vi "Robot Global Data.vi"() -> ()   [LabVIEW 2013]
doc: "This global VI can contain as many global variables as you need. Place a control on the panel, give it a good name. To read or write to it from a VI, drag the icon to the diagram of that VI. You can also drag from the project. Click on the node to change which global you access. You shouldn't have multiple locations writing to a global or it will cause a race-condition."
uses:
  <vilib>/Rock Robotics/WPI/Camera/WPI_CameraImageSize.ctl
  <vilib>/Rock Robotics/WPI/DriverStation/WPI_DriverStationRobotMode2.ctl
  Systems/DriverStation/DriverStation.lvclass
  Systems/Shifter/Shifter.lvclass
  Systems/GrabberArms/GrabberArms.lvclass
  Systems/GrabberWheels/GrabberWheels.lvclass
  Systems/Catapult/Catapult.lvclass
  Systems/Compressor/Compressor.lvclass
  Systems/DriveMotors/DriveMotors.lvclass
  Systems/Blocker/Blocker.lvclass
panel:
  out "Low Goal Auto":bool
  out "Catapult Auto":bool
  out "Block Auto":bool
  in  "Power":dbl
  in  "Time to Drive":u32
  out "Trim Left(T) or Right(F)":bool
  in  "Trim":dbl
  in  "Distance to Travel":dbl
  out "AutoMode: Drive Forward and Shoot":bool
  out "Blocker Enabled":bool=TRUE
  out "Catapult Enabled":bool=TRUE
  out "Shifter Enabled":bool=TRUE
  out "Grabber Wheels Enabled":bool=TRUE
  out "Grabber Arms Enabled":bool=TRUE
  out "DML Enabled":bool=TRUE
  out "DMR Enabled":bool=TRUE
  in  "Blocker":refnum<class "Blocker.lvclass">
  out "DMR":refnum<class "DriveMotors.lvclass">
  out "DML":refnum<class "DriveMotors.lvclass">
  in  "Compressor":refnum<class "Compressor.lvclass">
  in  "Catapult":refnum<class "Catapult.lvclass">
  in  "GrabberWheels":refnum<class "GrabberWheels.lvclass">
  in  "GrabberArms":refnum<class "GrabberArms.lvclass">
  in  "Shifter":refnum<class "Shifter.lvclass">
  in  "DriverStation":refnum<class "DriverStation.lvclass">
  in  "Robot Mode":T1
  in  "LED toggle rate (ms)":u32=20
  in  "image size":T2=enum."320x240"
  in  "Enable Vision":bool
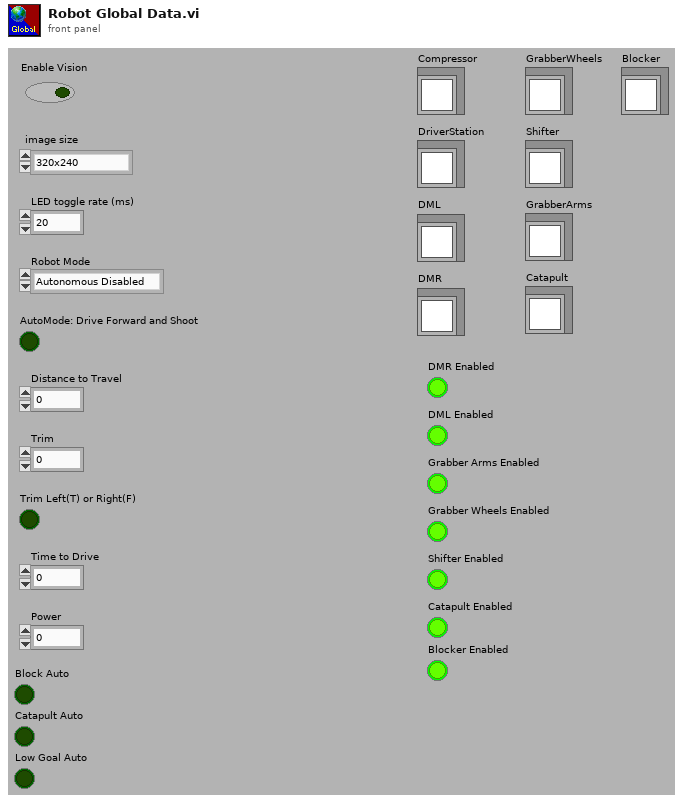
[diagram p1: front panel]
types:
  T1 = typedef "WPI_DriverStationRobotMode2.ctl" = enum16{"Autonomous Disabled", "Autonomous Enabled", "Teleop Disabled", "Teleop Enabled", "Timeout", "Finish", "Test Disabled", "Test Enabled"}
  T2 = typedef "WPI_CameraImageSize.ctl" = enum16{"640x480", "320x240", "160x120"}
diagram:
